vi "Write_Characters_no_warn.vi"(3 "append to file? (new file:F)":bool, 4 "character string":string, 5 "file path (dialog if empty)":path) -> (2 "new file path (Not A Path if cancelled)":path)   [LabVIEW 2010]
doc: "Writes a character string to a new byte stream file or appends the string to an existing file. The VI opens or creates the file beforehand and closes it afterwards.\n\nfile path is the path name of the file. If file path is empty (default value) or is Not A Path, the VI displays a File dialog box from which you can select a file. Error 43 occurs if the user cancels the dialog. \n\ncharacter string is the data the VI writes to the file.\n\nappend to file? Set to TRUE if you want to append the data to a existing file; you can also set it TRUE to write to a new file. Set to FALSE (default value) if you want to write the data to a new file or to replace an existing file.\n\nnew file path is the path of the file to which the VI wrote data. You can use this output to determine the path of a file that you open using dialog. new file path returns Not A Path if the user selects Cancel from the dialog box."
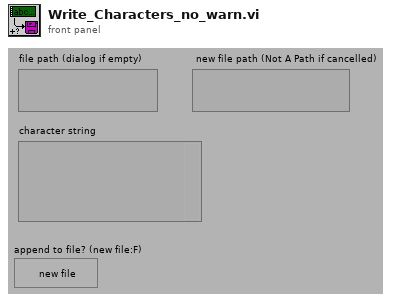
[diagram p1: front panel]
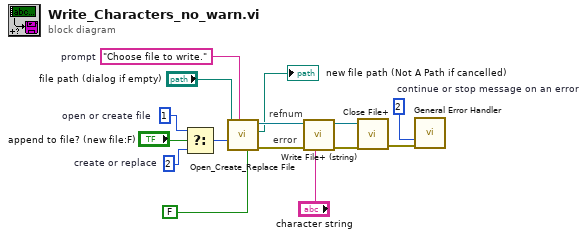
[diagram p0: block diagram]
diagram:
  w4 = i16 2  # create or replace
  w13 = 2  # continue or stop message on an error
  w10 = "Choose file to write."  # prompt
  w7 = i16 1  # open or create file
  # "error"
  # "refnum"
  n1 = Select(t=w7, s="append to file? (new file:F)", f=w4) -> (s? t:f=w9:i16)
  n2 = call <vilib>:"Open_Create_Replace File.vi"("advisory dialog? (display:T)"=FALSE, "prompt"=w10, "function (open:0)"=w9, "file path"="file path (dialog if empty)") -> ("error out"=w14:errorcluster, "new file path"=→"new file path (Not A Path if cancelled)":path, "refnum"=w3:refnum<file>)  [unwired: 4 in, 1 out]
  n3 = call <vilib>:"Write File+ (string).vi"("string"="character string", "error in (no error)"=w14, "refnum"=w3) -> ("error out"=w12:errorcluster, "dup refnum"=w11:refnum<file>)  [unwired: 4 in, 1 out]
  n4 = call <vilib>:"Close File+.vi"("error in (no error)"=w12, "refnum"=w11) -> ("error out"=w8:errorcluster)  [unwired: 3 in, 2 out]
  n5 = call <vilib>:"General Error Handler.vi"("type of dialog (OK msg:1)"=w13, "error in (no error)"=w8) -> ()  [unwired: 9 in, 5 out]
